vi "Uploader.vi"() -> ()   [LabVIEW 2011]
uses:
  Typedef/ManUIref.ctl
  CAN FD.lvlib
panel:
  in  "Close":bool
  in  "UpdateFW":bool
  in  "DevInfo":bool
  in  "Open":bool
  in  "Index":u32(ring) caption="索引" items=["0", "1", "2", "3", "4", "5", "6", "7", "8"]
  in  "Type":u32(ring)=41 caption="CAN卡型号" items=["USBCANFD-200U"=41, "USBCANFD-100U"=42]
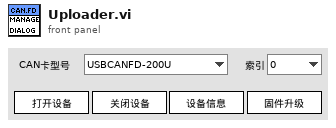
[diagram p1: front panel]
types:
  T1 = typedef "CAN FD.lvlib/ManUIref.ctl" = cluster{"Type":refnum<vi>, "Index":refnum<vi>, "Open":refnum<vi>, "Close":refnum<vi>, "DevInfo":refnum<vi>, "Update":refnum<vi>}
  T2 = cluster{"Type":u32, "Index":u32, "DeviceOpen":bool, "Ch0Start":bool, "Ch1Start":bool}
  T3 = cluster{"Terminal":u32, "Param":cluster{"abitbaud":u32, "dbitbaud":u32, "CustomBaud":bool, "CustomBd":string, "Mode":u8}}
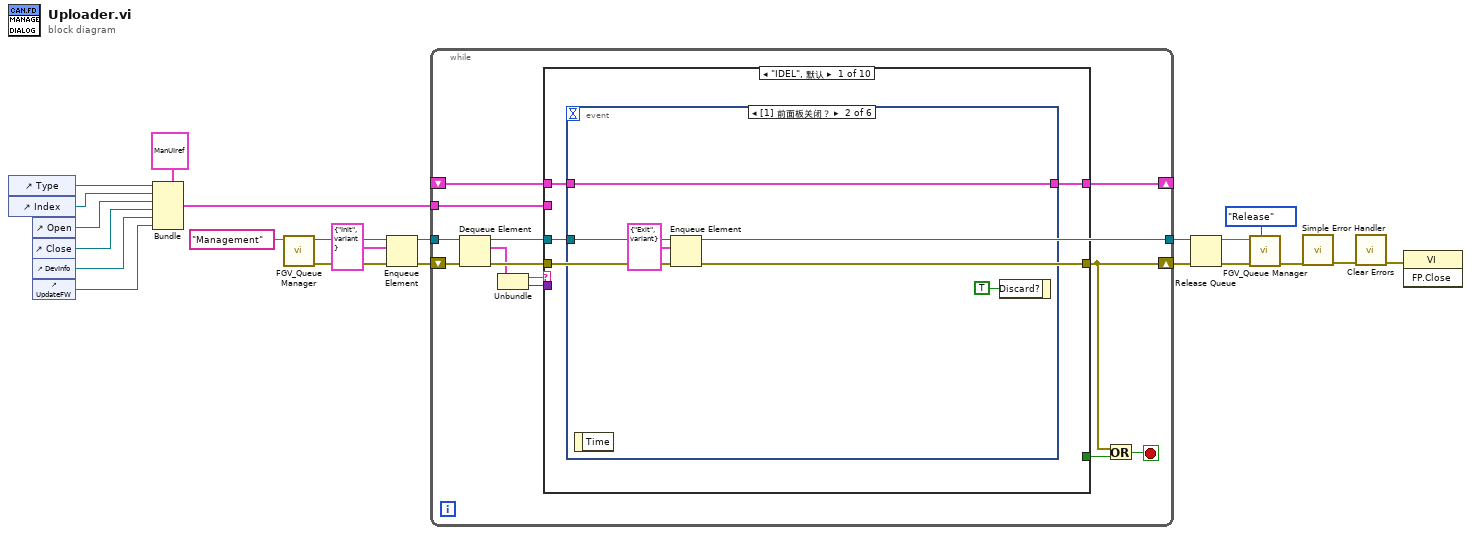
[diagram p0: block diagram]
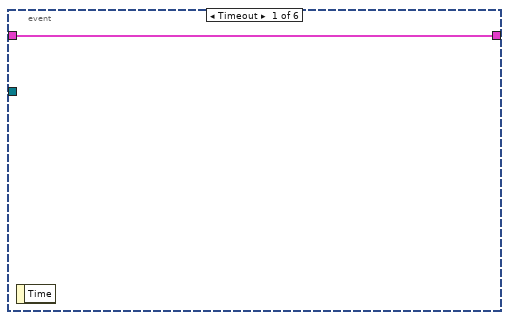
[diagram p2: hidden frame]
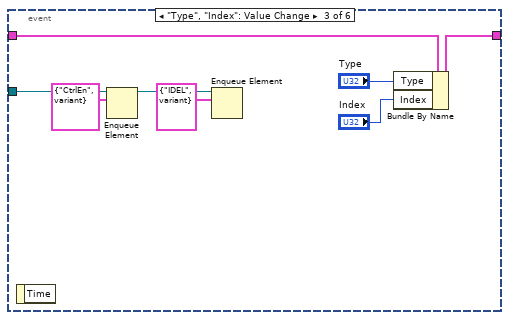
[diagram p3: hidden frame]
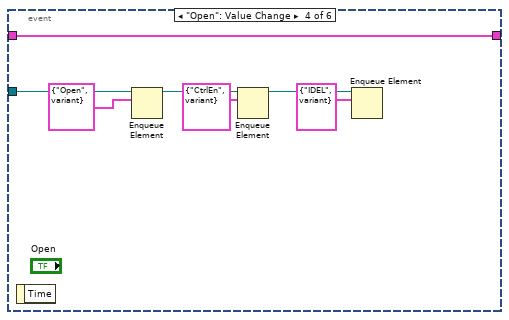
[diagram p4: hidden frame]
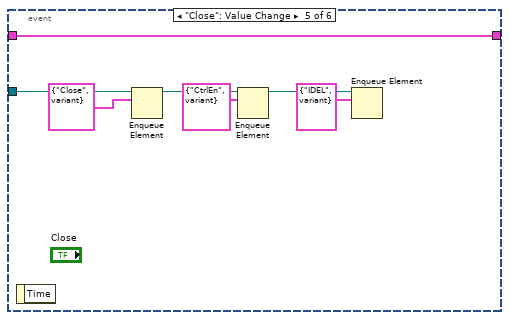
[diagram p5: hidden frame]
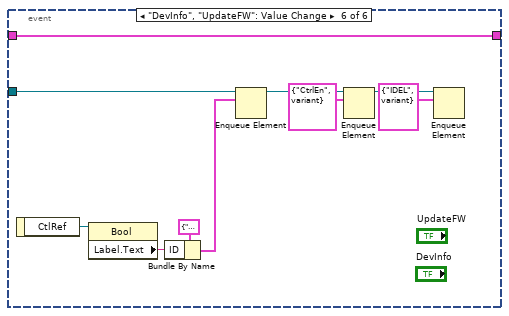
[diagram p6: hidden frame]
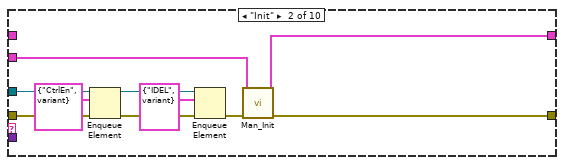
[diagram p7: hidden frame]
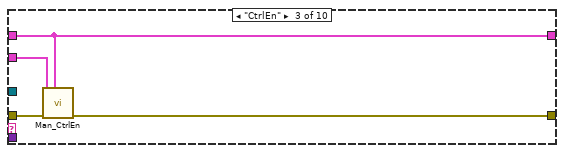
[diagram p8: hidden frame]
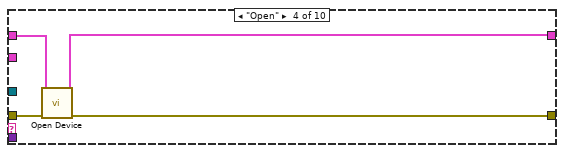
[diagram p9: hidden frame]
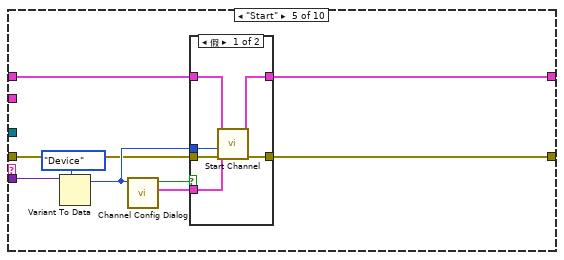
[diagram p10: hidden frame]
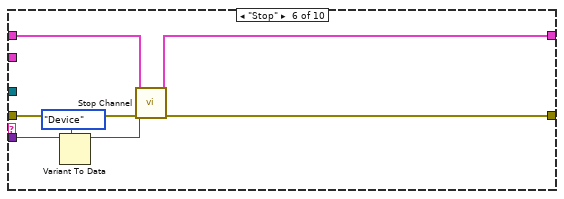
[diagram p12: hidden frame]
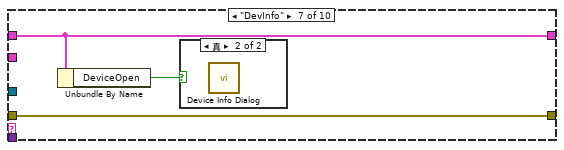
[diagram p13: hidden frame]
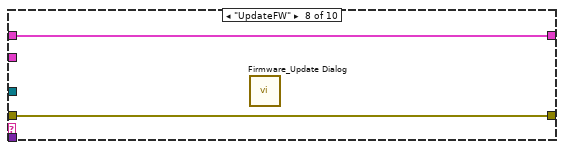
[diagram p15: hidden frame]
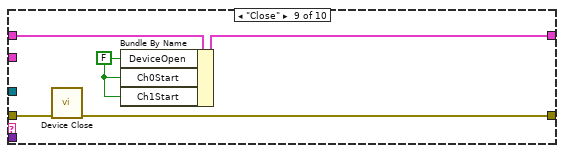
[diagram p16: hidden frame]
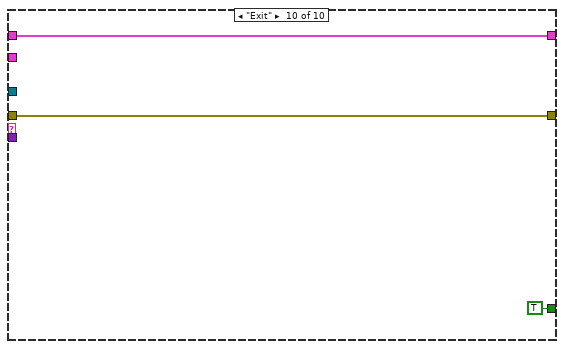
[diagram p17: hidden frame]
diagram:
  n1 = control-ref of="Type"() -> (w12:refnum<vi>)
  n2 = control-ref of="Index"() -> (w11:refnum<vi>)
  n3 = control-ref of="Open"() -> (w10:refnum<vi>)
  n4 = control-ref of="Close"() -> (w9:refnum<vi>)
  n5 = control-ref of="DevInfo"() -> (w2:refnum<vi>)
  n6 = control-ref of="UpdateFW"() -> (w1:refnum<vi>)
  n7 = Bundle(cluster=T1 {"Type"=refnum, "Index"=refnum, "Open"=refnum, "Close"=refnum, "DevInfo"=refnum, "Update"=refnum} ("ManUIref"), "Type"=w12, "Index"=w11, "Open"=w10, "Close"=w9, "DevInfo"=w2, "Update"=w1) -> (w7:T1)
  n8 = call "FGV_Queue Manager.vi"("Name"="Management") -> ("error out"=w21:errorcluster, "Queue"=w22:refnum<queue>)  [unwired: 8 in, 1 out]
  n9 = Enqueue Element(queue=w22, element=cluster{"ID":string, "Data":variant} {"ID"="Init", "Data"=variant} ("元素"), error in (no error)=w21) -> (queue out=w17:refnum<queue>, error out=w18:errorcluster)  [unwired: 1 in, 1 out]
  n10 = while {
    tunnel: w17 -> [w34]
    tunnel: [w25] -> w15
    shift-right: [w26] -> w16
    shift-left: w18 -> [w35]
    tunnel: w7 -> [w27]
    shift-right: [w24] -> _
    shift-left: _ -> [w23]
    stop <- w29 stop-if-true
    n11 = Dequeue Element(queue=w34, error in (no error)=w35) -> (queue out=w25:refnum<queue>, element=w28:cluster{"ID":string, "Data":variant}, error out=w31:errorcluster)  [unwired: 1 in, 1 out]
    n12 = Unbundle(w28) -> ("ID"=w33:string, "Data"=w32:variant)
    n13 = case shown="\"IDEL\", 默认" w33 {
      tunnel: w32 -> [_ _ _ _ w103 w118 _ _ _ _]
      tunnel: [_ _ _ _ _ _ _ _ _ TRUE] -> w30
      tunnel: [w39 w84 w89 w93 w95 w115 w121 w122 w127 w130] -> w26
      tunnel: w31 -> [w39 w79 w90 w94 w96 w116 w121 w122 w128 w130]
      tunnel: w25 -> [w38 w80 _ _ _ _ _ _ _ _]
      tunnel: w27 -> [_ w82 w88 _ _ _ _ _ _ _]
      tunnel: [w37 w83 w87 w91 w98 w113 w120 w123 w124 w129] -> w24
      tunnel: w23 -> [w36 _ w87 w92 w97 w114 w120 w123 w126 w129]
      frame "IDEL", Default {
        n14 = event shown="[1] 前面板关闭？" {
          selector: _ -> [_ _ _ _ _ _]
          dyn-events: _ -> [_ _ _ _ _ _]
          timeout: _ -> [_ _ _ _ _ _]
          tunnel: w38 -> [_ w43 w49 w57 w64 w69]
          tunnel: [w40 w41 w45 w59 w66 w76] -> w37
          tunnel: w36 -> [w40 w41 w48 w59 w66 w76]
          event Timeout {
            n15 = event-data() -> ()  [unwired: 1 in, 1 out]
          }
          event Panel Close? {
            n16 = event-data() -> ()  [unwired: 1 in, 1 out]
            n17 = Enqueue Element(queue=w43, element=cluster{"ID":string, "Data":variant} {"ID"="Exit", "Data"=variant} ("元素")) -> ()  [unwired: 2 in, 3 out]
            n18 = event-data("Discard?"=TRUE ("放弃？")) -> ()  [unwired: 1 in, 1 out]
          }
          event "Type", "Index": Value Change {
            n19 = event-data() -> ()  [unwired: 1 in, 1 out]
            n20 = Enqueue Element(queue=w49, element=cluster{"ID":string, "Data":variant} {"ID"="CtrlEn", "Data"=variant} ("元素")) -> (queue out=w50:refnum<queue>)  [unwired: 2 in, 2 out]
            n21 = Enqueue Element(queue=w50, element=cluster{"ID":string, "Data":variant} {"ID"="IDEL", "Data"=variant} ("元素")) -> ()  [unwired: 2 in, 3 out]
            n22 = Bundle By Name(cluster=w48, "Type"="Type", "Index"="Index") -> (w45:T2)
          }
          event "Open": Value Change {
            n23 = event-data() -> ()  [unwired: 1 in, 1 out]
            n24 = Enqueue Element(queue=w57, element=cluster{"ID":string, "Data":variant} {"ID"="Open", "Data"=variant} ("元素")) -> (queue out=w54:refnum<queue>)  [unwired: 2 in, 2 out]
            n25 = Enqueue Element(queue=w54, element=cluster{"ID":string, "Data":variant} {"ID"="CtrlEn", "Data"=variant} ("元素")) -> (queue out=w53:refnum<queue>)  [unwired: 2 in, 2 out]
            n26 = Enqueue Element(queue=w53, element=cluster{"ID":string, "Data":variant} {"ID"="IDEL", "Data"=variant} ("元素")) -> ()  [unwired: 2 in, 3 out]
          }
          event "Close": Value Change {
            n27 = event-data() -> ()  [unwired: 1 in, 1 out]
            n28 = Enqueue Element(queue=w64, element=cluster{"ID":string, "Data":variant} {"ID"="Close", "Data"=variant} ("元素")) -> (queue out=w61:refnum<queue>)  [unwired: 2 in, 2 out]
            n29 = Enqueue Element(queue=w61, element=cluster{"ID":string, "Data":variant} {"ID"="CtrlEn", "Data"=variant} ("元素")) -> (queue out=w60:refnum<queue>)  [unwired: 2 in, 2 out]
            n30 = Enqueue Element(queue=w60, element=cluster{"ID":string, "Data":variant} {"ID"="IDEL", "Data"=variant} ("元素")) -> ()  [unwired: 2 in, 3 out]
          }
          event "DevInfo", "UpdateFW": Value Change {
            n31 = event-data() -> ("CtlRef"=w72:refnum<vi>)  [unwired: 1 in]
            n32 = property class="Bool"(reference=w72) -> ("Label.Text"=w70:string)  [unwired: 1 in, 2 out]
            n33 = Bundle By Name(cluster=cluster{"ID":string, "Data":variant} {"ID"="", "Data"=variant} ("元素"), "ID"=w70) -> (w67:cluster{"ID":string, "Data":variant})
            n34 = Enqueue Element(queue=w69, element=w67) -> (queue out=w68:refnum<queue>)  [unwired: 2 in, 2 out]
            n35 = Enqueue Element(queue=w68, element=cluster{"ID":string, "Data":variant} {"ID"="CtrlEn", "Data"=variant} ("元素")) -> (queue out=w73:refnum<queue>)  [unwired: 2 in, 2 out]
            n36 = Enqueue Element(queue=w73, element=cluster{"ID":string, "Data":variant} {"ID"="IDEL", "Data"=variant} ("元素")) -> ()  [unwired: 2 in, 3 out]
          }
        }
      }
      frame "Init" {
        n37 = Enqueue Element(queue=w80, element=cluster{"ID":string, "Data":variant} {"ID"="CtrlEn", "Data"=variant} ("元素"), error in (no error)=w79) -> (queue out=w78:refnum<queue>, error out=w77:errorcluster)  [unwired: 1 in, 1 out]
        n38 = Enqueue Element(queue=w78, element=cluster{"ID":string, "Data":variant} {"ID"="IDEL", "Data"=variant} ("元素"), error in (no error)=w77) -> (error out=w85:errorcluster)  [unwired: 1 in, 2 out]
        n39 = call "Man_Init.vi"("error in (no error)"=w85, "ManUIref"=w82) -> ("error out"=w84:errorcluster, "DevState"=w83:T2)  [unwired: 8 in]
      }
      frame "CtrlEn" {
        n40 = call "Man_CtrlEn.vi"("DevState"=w87, "error in (no error)"=w90, "ManUIref"=w88) -> ("error out"=w89:errorcluster)  [unwired: 8 in]
      }
      frame "Open" {
        n41 = call "Open Device.vi"("error in (no error)"=w94, "DevState"=w92) -> ("error out"=w93:errorcluster, "DevState out"=w91:T2)  [unwired: 8 in]
      }
      frame "Start" {
        n42 = Variant To Data(type=enum16{"Device", "Ch0", "Ch1"}."Device", Variant=w103) -> (data=w99:enum16{"Device", "Ch0", "Ch1"})  [unwired: 1 in, 1 out]
        n43 = call "Channel Config Dialog.vi"("Type"=w99) -> ("Param"=w100:T3, "Cancel"=w101:bool)  [unwired: 8 in, 1 out]
        n44 = case shown="假" w101 {
          tunnel: w100 -> [w104 _]
          tunnel: w99 -> [w105 _]
          tunnel: [w106 w111] -> w98
          tunnel: w97 -> [w107 w111]
          tunnel: w96 -> [w109 w110]
          tunnel: [w108 w110] -> w95
          frame False {
            n45 = call "Start Channel.vi"("error in (no error)"=w109, "ChannelType"=w105, "Param"=w104, "DevState"=w107) -> ("error out"=w108:errorcluster, "DevState out"=w106:T2)  [unwired: 6 in]
          }
          frame True {
          }
        }
      }
      frame "Stop" {
        n46 = Variant To Data(type=enum16{"Device", "Ch0", "Ch1"}."Device", Variant=w118) -> (data=w112:enum16{"Device", "Ch0", "Ch1"})  [unwired: 1 in, 1 out]
        n47 = call "Stop Channel.vi"("error in (no error)"=w116, "ChannelType"=w112, "DevState"=w114) -> ("error out"=w115:errorcluster, "DevState out"=w113:T2)  [unwired: 7 in]
      }
      frame "DevInfo" {
        n48 = Unbundle By Name(w120) -> ("DeviceOpen"=w119:bool)
        n49 = case shown="真" w119 {
          frame False {
          }
          frame True {
            n50 = call "Device Info Dialog.vi"() -> ()  [unwired: 12 in]
          }
        }
      }
      frame "UpdateFW" {
        n51 = call "Firmware_Update Dialog.vi"() -> ()  [unwired: 12 in]
      }
      frame "Close" {
        w125 = FALSE ("DeviceOpen")
        n52 = call "Device Close.vi"("error in (no error)"=w128) -> ("error out"=w127:errorcluster)  [unwired: 10 in]
        n53 = Bundle By Name(cluster=w126, "DeviceOpen"=w125, "Ch0Start"=w125, "Ch1Start"=w125) -> (w124:T2)
      }
      frame "Exit" {
      }
    }
    n54 = Or(x=w26, y=w30) -> (x .or. y?=w29:bool)
  }
  n55 = Release Queue(queue=w15, error in (no error)=w16) -> (queue name=w5:string, error out=w6:errorcluster)  [unwired: 1 in, 1 out]
  n56 = call "FGV_Queue Manager.vi"("Methods"=enum16{"Init", "Get", "Release", "Destroy"}."Release", "error in (no error)"=w6, "Name"=w5) -> ("error out"=w4:errorcluster)  [unwired: 6 in, 2 out]
  n57 = call <vilib>:"Simple Error Handler.vi"("error in (no error)"=w4) -> ("error out"=w14:errorcluster)  [unwired: 4 in, 4 out]
  n58 = call <vilib>:"Clear Errors.vi"("error in (no error)"=w14) -> ("error out"=w13:errorcluster)  [unwired: 6 in]
  n59 = invoke class="VI" method="FP.Close"(error in=w13) -> ()  [unwired: 2 in, 3 out]
